vi "Notify.vi"(8 "error in (no error)":errorcluster, 9 "Value":variant, 11 "ISubject in":refnum<class "ISubject.lvclass">) -> (0 "error out":errorcluster, 3 "ISubject out":refnum<class "ISubject.lvclass">)   [LabVIEW 2015, in "Observer.lvlib" / "ISubject.lvclass"]
uses:
  ISubject.lvclass
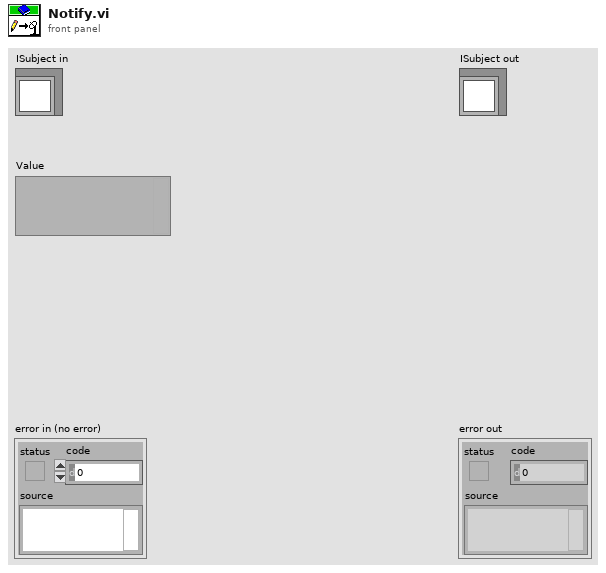
[diagram p1: front panel]
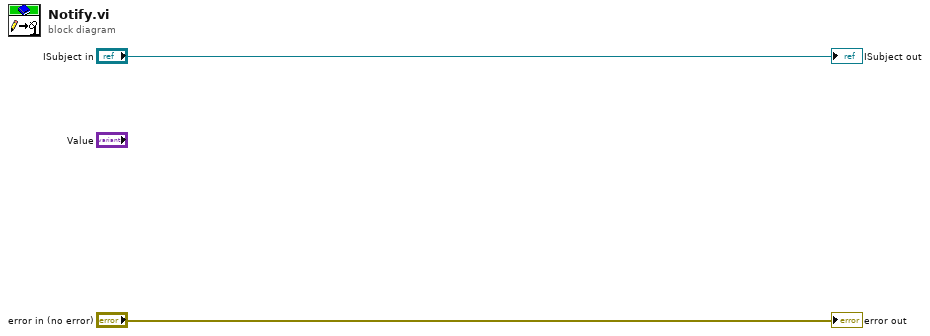
[diagram p0: block diagram]
diagram:
  "error out" <- "error in (no error)"
  "ISubject out" <- "ISubject in"
